vi "GetObject_LeftSR.vi"(5 "UID":i32, 6 "error in":errorcluster, 9 "VI Interpreter in":refnum<class "VI Interpreter.lvclass">) -> (0 "error out":errorcluster, 1 "found":bool, 3 "VI Interpreter out":refnum<class "VI Interpreter.lvclass">, 4 "SR":refnum<class "LeftShiftRegister.lvclass">)   [LabVIEW 2014, in "Raspberry Pi Compatible Compiler for LabVIEW.lvlib" / "VI Interpreter.lvclass"]
uses:
  VI Interpreter.lvclass
  LeftShiftRegister/LeftShiftRegister.lvclass
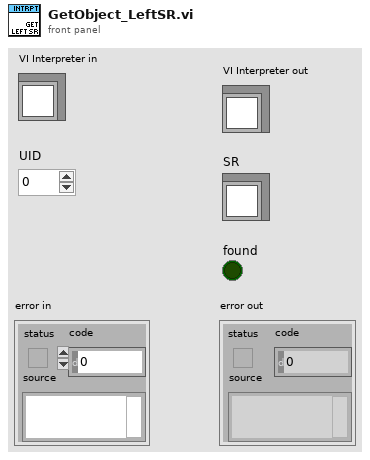
[diagram p1: front panel]
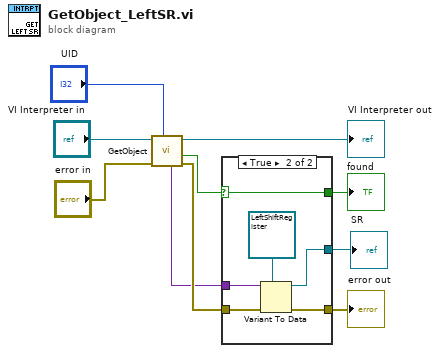
[diagram p0: block diagram]
diagram:
  n1 = call "GetObject.vi"("UID"="UID", "error in"="error in", "VI Interpreter in"="VI Interpreter in") -> ("error out"=w5:errorcluster, "found"=w3:bool, "VI Interpreter out"=→"VI Interpreter out":refnum<class "VI Interpreter.lvclass">, "value"=w4:variant)  [unwired: 3 in]
  n2 = case shown="True" w3 {
    selector: w3 -> [w12 w15]
    tunnel: [w11 w18] -> w6
    tunnel: w5 -> [w11 w17]
    tunnel: w4 -> [_ w16]
    tunnel: [w12 w15] -> w2
    tunnel: [_ w14] -> w1
    frame False {
    }
    frame True {
      n3 = Variant To Data(error in=w17, type=refnum<class "LeftShiftRegister.lvclass"> refnum ("Terminal"), Variant=w16) -> (data=w14:refnum<class "LeftShiftRegister.lvclass">, error out=w18:errorcluster)
    }
  }
  "error out" <- w6
  "SR" <- w1
  "found" <- w2
